vi "Simulation.vi"() -> ()   [LabVIEW 2017]
uses:
  Control/SimulationMainEnum.ctl
  Control/SimulationColorTypeEnum.ctl
panel:
  out "ErrorMsg":string
  out "Boolean":bool
  out "Incremento":dbl
  out "VelocidadFicha":dbl
  in  "TokenColor":T1
  out "Horizontal Pointer Slide":dbl(slide) scale=0.0..100.0
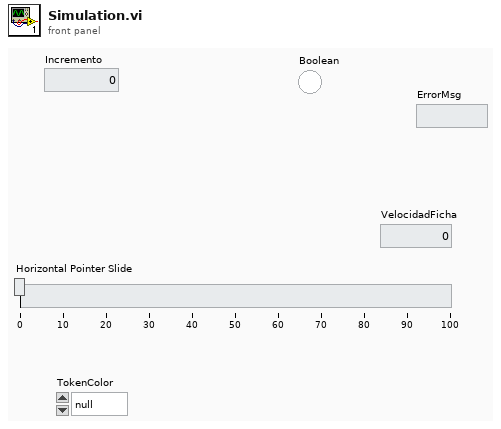
[diagram p1: front panel]
types:
  T1 = typedef "SimulationColorTypeEnum.ctl" = enum16{"null", "White", "Blue", "Red"}
  T2 = typedef "SimulationMainEnum.ctl" = enum16{"idle", "Simulation", "Error", "Stop"}
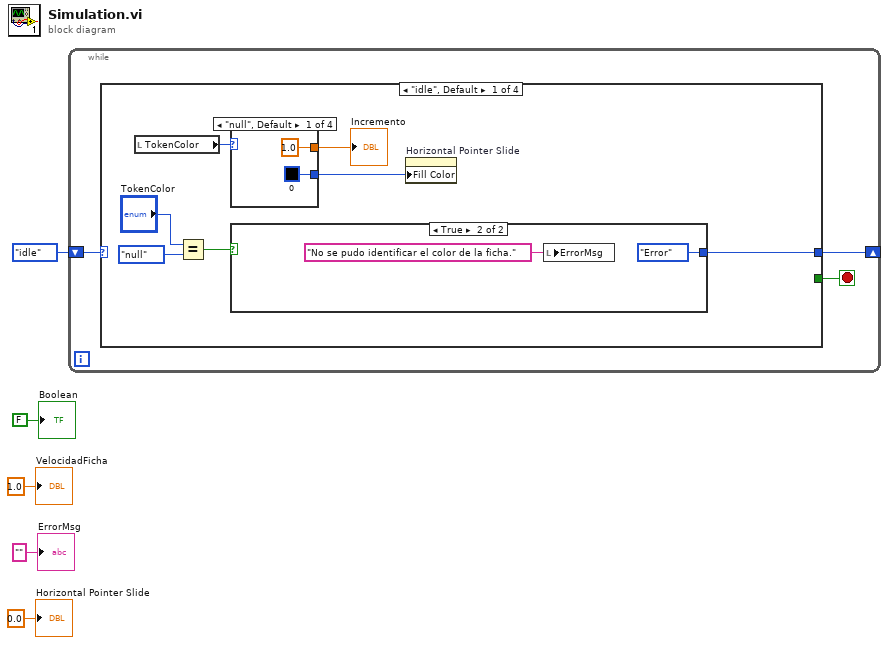
[diagram p0: block diagram]
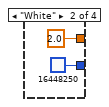
[diagram p2: hidden frame]
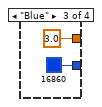
[diagram p3: hidden frame]
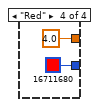
[diagram p4: hidden frame]
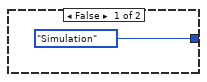
[diagram p5: hidden frame]
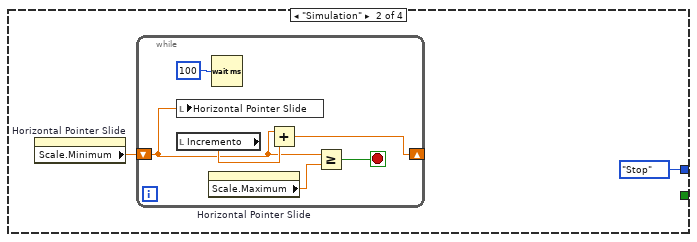
[diagram p6: hidden frame]
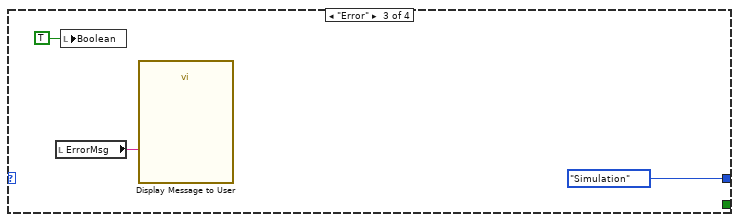
[diagram p7: hidden frame]
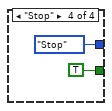
[diagram p8: hidden frame]
diagram:
  n1 = while {
    shift-right: [w7] -> _
    shift-left: SimulationMainEnum."idle" -> [w8]
    stop <- w6 stop-if-true
    n2 = case shown="\"idle\", Default" w8 {
      tunnel: [w12 SimulationMainEnum."Stop" SimulationMainEnum."Simulation" SimulationMainEnum."Stop"] -> w7
      tunnel: [_ _ _ TRUE] -> w6
      frame "idle", Default {
        n3 = local read "TokenColor"() -> (w11:T1)
        n4 = Equal?(x="TokenColor", y=SimulationColorTypeEnum."null") -> (x = y?=w13:bool)
        n5 = case shown="\"null\", Default" w11 {
          tunnel: [u32 0 ("Color Box") u32 16448250 ("Color Box") u32 16860 ("Color Box") u32 16711680 ("Color Box")] -> w10
          tunnel: [1.0 ("Incremento") 2.0 ("Incremento") 3.0 ("Incremento") 4.0 ("Incremento")] -> w9
          frame "null", Default {
          }
          frame "White" {
          }
          frame "Blue" {
          }
          frame "Red" {
          }
        }
        "Incremento" <- w9
        n6 = case shown="True" w13 {
          tunnel: [SimulationMainEnum."Simulation" SimulationMainEnum."Error"] -> w12
          frame False {
          }
          frame True {
            n7 = local write "ErrorMsg"("No se pudo identificar el color de la ficha." ("ErrorMsg")) -> ()
          }
        }
        n8 = property on="Horizontal Pointer Slide" class="Slide (strict)"("Fill Color"=w10) -> ()  [unwired: 2 in, 2 out]
      }
      frame "Simulation" {
        n9 = property on="Horizontal Pointer Slide" class="Slide (strict)"() -> ("Scale.Minimum"=w27:dbl)  [unwired: 2 in, 2 out]
        n10 = while {
          shift-right: [w33] -> _
          shift-left: w27 -> [w32]
          stop <- w31 stop-if-true
          n11 = local write "Horizontal Pointer Slide"(w32) -> ()
          n12 = local read "Incremento"() -> (w34:dbl)
          n13 = property on="Horizontal Pointer Slide" class="Slide (strict)"() -> ("Scale.Maximum"=w30:dbl)  [unwired: 2 in, 2 out]
          n14 = Wait (ms)(milliseconds to wait=u32 100) -> ()  [unwired: 1 out]
          n15 = Add(x=w32, y=w34) -> (x+y=w33:dbl)
          n16 = Greater Or Equal?(x=w32, y=w30) -> (x >= y?=w31:bool)
        }
      }
      frame "Error" {
        n17 = local read "ErrorMsg"() -> (w35:string)
        n18 = local write "Boolean"(TRUE ("Boolean")) -> ()
        n19 = call "Display Message to User"("Message"=w35) -> ()  [unwired: 9 in, 2 out]
      }
      frame "Stop" {
      }
    }
  }
  "VelocidadFicha" <- 1.0 ("VelocidadFicha")
  "Boolean" <- FALSE ("Boolean")
  "Horizontal Pointer Slide" <- 0.0 ("Horizontal Pointer Slide")
  "ErrorMsg" <- "" ("ErrorMsg")
